vi "Init.vi"(8 "error in (no error)":errorcluster, 10 "Channel":i16, 11 "TrialBasedExperiment in":refnum<class "MoviesExperiment.lvclass">) -> (0 "error out":errorcluster, 3 "TrialBasedExperiment out":refnum<class "MoviesExperiment.lvclass">)   [LabVIEW 2012, in "MoviesExperiment.lvclass"]
uses:
  MoviesExperiment.lvclass
  Trial Based Experiment Statechart/PassiveExperiment/PassiveExperiment.lvclass
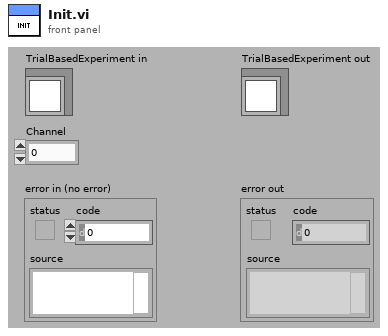
[diagram p1: front panel]
types:
  T1 = cluster{"Intertrial":dbl, "AcquireFixation":dbl, "HoldFixation":dbl, "DelayPeriod":dbl, "ResponsePeriod":dbl}
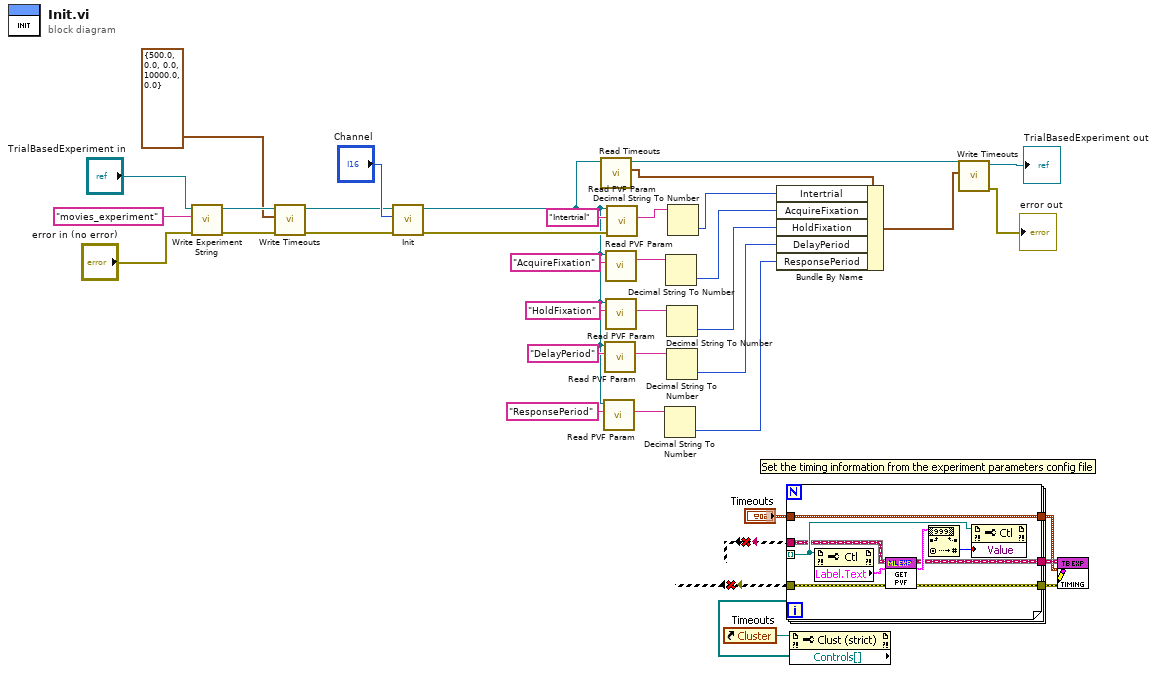
[diagram p0: block diagram]
diagram:
  n1 = call-dynamic "Write Experiment String.vi"("error in (no error)"="error in (no error)", "Experiment String"="movies_experiment", "TrialBasedExperiment in"="TrialBasedExperiment in") -> ("error out"=w28:errorcluster, "TrialBasedExperiment out"=w29:refnum<class "MoviesExperiment.lvclass">)  [unwired: 7 in]
  n2 = call-dynamic "Write Timeouts.vi"("error in (no error)"=w28, "Timeouts"=T1 {"Intertrial"=500.0, "AcquireFixation"=0.0, "HoldFixation"=0.0, "DelayPeriod"=10000.0, "ResponsePeriod"=0.0}, "TrialBasedExperiment in"=w29) -> ("error out"=w26:errorcluster, "TrialBasedExperiment out"=w23:refnum<class "MoviesExperiment.lvclass">)  [unwired: 7 in]
  n3 = call-parent "Init.vi"("error in (no error)"=w26, "Channel"="Channel", "TrialBasedExperiment in"=w23) -> ("error out"=w19:errorcluster, "TrialBasedExperiment out"=w14:refnum<class "MoviesExperiment.lvclass">)  [unwired: 7 in]
  n4 = call-dynamic "Read Timeouts.vi"("TrialBasedExperiment in"=w14) -> ("Timeouts"=w22:T1, "TrialBasedExperiment out"=w20:refnum<class "MoviesExperiment.lvclass">)  [unwired: 8 in, 1 out]
  n5 = call-dynamic "Read PVF Param.vi"("Param Name"="ResponsePeriod", "MatlabExperiment in"=w14) -> ("Param Value"=w8:string)  [unwired: 7 in, 2 out]
  n6 = call-dynamic "Read PVF Param.vi"("Param Name"="DelayPeriod", "MatlabExperiment in"=w14) -> ("Param Value"=w7:string)  [unwired: 7 in, 2 out]
  n7 = call-dynamic "Read PVF Param.vi"("Param Name"="AcquireFixation", "MatlabExperiment in"=w14) -> ("Param Value"=w9:string)  [unwired: 7 in, 2 out]
  n8 = call-dynamic "Read PVF Param.vi"("Param Name"="HoldFixation", "MatlabExperiment in"=w14) -> ("Param Value"=w6:string)  [unwired: 7 in, 2 out]
  n9 = call-dynamic "Read PVF Param.vi"("error in (no error)"=w19, "Param Name"="Intertrial", "MatlabExperiment in"=w14) -> ("Param Value"=w12:string)  [unwired: 6 in, 2 out]
  n10 = Decimal String To Number(string=w8) -> (number=w3:i32)  [unwired: 2 in, 1 out]
  n11 = Decimal String To Number(string=w9) -> (number=w10:i32)  [unwired: 2 in, 1 out]
  n12 = Decimal String To Number(string=w6) -> (number=w5:i32)  [unwired: 2 in, 1 out]
  n13 = Decimal String To Number(string=w7) -> (number=w4:i32)  [unwired: 2 in, 1 out]
  n14 = Decimal String To Number(string=w12) -> (number=w11:i32)  [unwired: 2 in, 1 out]
  n15 = Bundle By Name(cluster=w22, "Intertrial"=w11, "AcquireFixation"=w10, "HoldFixation"=w5, "DelayPeriod"=w4, "ResponsePeriod"=w3) -> (w21:T1)
  n16 = call-dynamic "Write Timeouts.vi"("Timeouts"=w21, "TrialBasedExperiment in"=w20) -> ("error out"=→"error out":errorcluster, "TrialBasedExperiment out"=→"TrialBasedExperiment out":refnum<class "MoviesExperiment.lvclass">)  [unwired: 8 in]
